vi "ArrayOfPossibleDevices.vi"() -> (3 "Array of device types":refnum<class "GenericDevice.lvclass">[](array[class]))   [LabVIEW 2023]
uses:
  Classes/GenericDevice/GenericDevice.lvclass
  Classes/Mono/Monochromator.lvclass
  Classes/SCD/SCD.lvclass
  Classes/CCD/CCD.lvclass
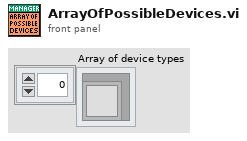
[diagram p1: front panel]
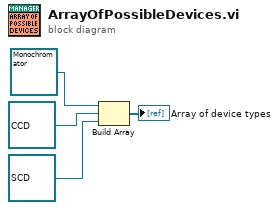
[diagram p0: block diagram]
diagram:
  n1 = Build Array(refnum<class "Monochromator.lvclass"> refnum ("Monochromator.lvclass"), refnum<class "CCD.lvclass"> refnum ("CCD.lvclass"), refnum<class "SCD.lvclass"> refnum ("SCD.lvclass")) -> (→"Array of device types":refnum<class "GenericDevice.lvclass">[])
